vi "acquire.vi"(8 "error in (no error)":errorcluster, 11 "Measurement in":refnum<class "Measurement.lvclass">) -> (0 "error out":errorcluster, 3 "Measurement out":refnum<class "Measurement.lvclass">)   [LabVIEW 2017, in "Measurement.lvclass"]
doc: "Acquire data for a measurement"
uses:
  Measurement.lvclass
  measurement_result/MeasurementResult.lvclass
  Measurement.lvclass/Measurement.ctl
  hardware/Hardware.lvclass
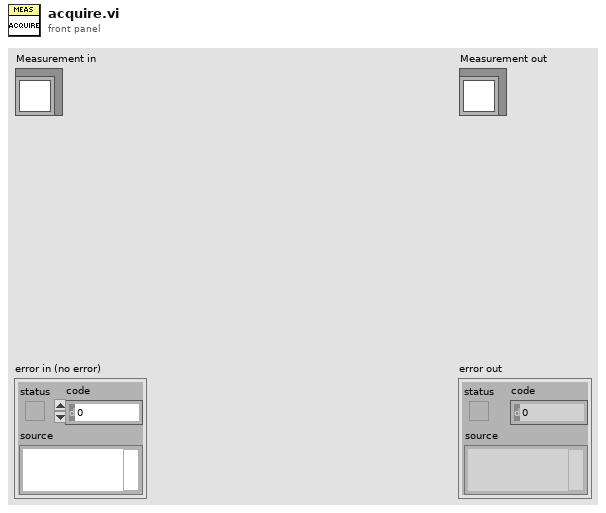
[diagram p1: front panel]
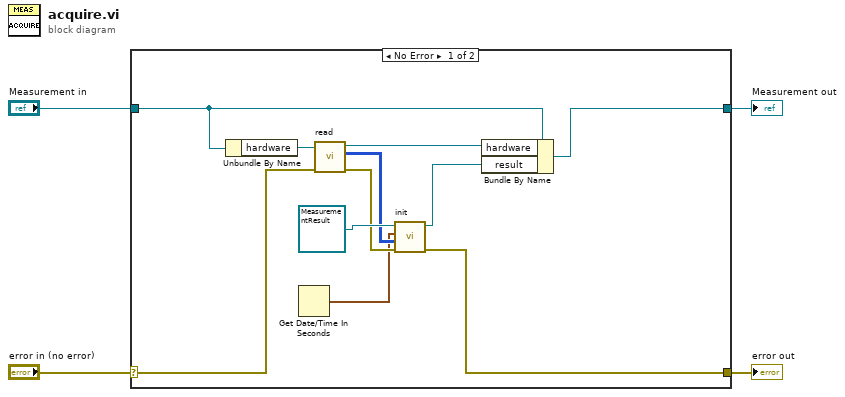
[diagram p0: block diagram]
diagram:
  n1 = case shown="No Error" "error in (no error)" {
    selector: "error in (no error)" -> [w11 w17]
    tunnel: [w7 w17] -> w3
    tunnel: [w13 w16] -> w1
    tunnel: "Measurement in" -> [w14 w16]
    frame No Error {
      n2 = Unbundle By Name(w14) -> ("hardware"=w15:refnum<class "Hardware.lvclass">)
      n3 = Get Date/Time In Seconds() -> (seconds since 1Jan1904=w5:timestamp)
      n4 = call-dynamic "read.vi"("error in (no error)"=w11, "Hardware in"=w15) -> ("error out"=w9:errorcluster, "outputs"=w6:u16[][], "Hardware out"=w12:refnum<class "Hardware.lvclass">)  [unwired: 7 in]
      n5 = call-dynamic "init.vi"("error in (no error)"=w9, "inputs"=w6, "time_stamp"=w5, "MeasurementResult in"=refnum<class "MeasurementResult.lvclass"> refnum ("MeasurementResult.lvclass")) -> ("error out"=w7:errorcluster, "MeasurementResult out"=w8:refnum<class "MeasurementResult.lvclass">)  [unwired: 6 in]
      n6 = Bundle By Name(cluster=w14, "hardware"=w12, "result"=w8) -> (w13:refnum<class "Measurement.lvclass">)
    }
    frame Error {
    }
  }
  "error out" <- w3
  "Measurement out" <- w1
